vi "Close Instrument.vi"(8 "error in (no error)":errorcluster {"code" format="%.0x"}, 11 "NI Switch.lvclass":refnum<class "NI Switch.lvclass">) -> (0 "error out":errorcluster, 3 "NI Switch.lvclass 2":refnum<class "NI Switch.lvclass">)   [LabVIEW 2010, in "NI Switch.lvclass"]
uses:
  NI Switch.lvclass
  NI Switch.lvclass/NI Switch.ctl
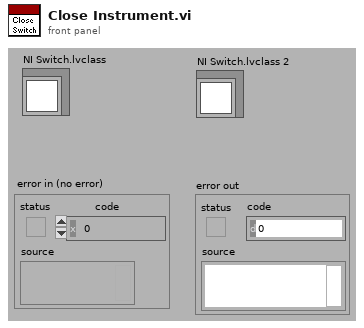
[diagram p1: front panel]
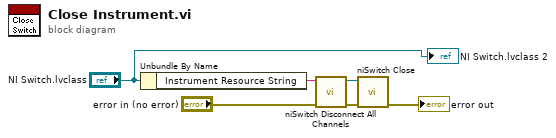
[diagram p0: block diagram]
diagram:
  n1 = Unbundle By Name("NI Switch.lvclass") -> ("Instrument Resource String"=w2:string)
  n2 = call <instrlib>:"niSwitch Disconnect All Channels.vi"("error in (no error)"="error in (no error)", "instrument handle"=w2) -> ("error out"=w4:errorcluster, "instrument handle out"=w3:refnum<k15>)  [unwired: 8 out]
  n3 = call <instrlib>:"niSwitch Close.vi"("error in (no error)"=w4, "instrument handle"=w3) -> ("error out"=→"error out":errorcluster)  [unwired: 2 in, 7 out]
  "NI Switch.lvclass 2" <- "NI Switch.lvclass"
